vi "DP-Coerce Frequency.vi"(9 "Npts":i32, 10 "Sampling rate (Hz)":dbl, 11 "Frequency (kHz)":dbl[](array[numeric])) -> (1 "Npts":i32, 2 "Sampling rate (Hz)":dbl, 3 "Coerced Frequency (kHz)":dbl[](array[numeric]))   [LabVIEW 2020]
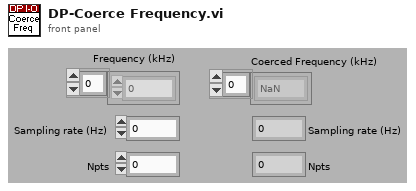
[diagram p1: front panel]
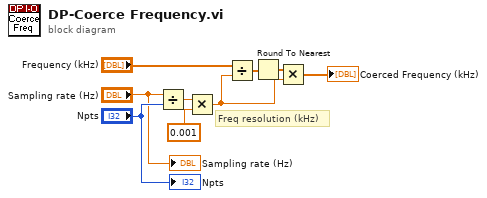
[diagram p0: block diagram]
diagram:
  # "Freq resolution (kHz)"
  n1 = Divide(x="Sampling rate (Hz)", y="Npts") -> (x/y=w9:dbl)
  n2 = Multiply(x=w9, y=0.001) -> (x*y=w6:dbl)
  n3 = Divide(x="Frequency (kHz)", y=w6) -> (x/y=w8:dbl[])
  n4 = Round To Nearest(number=w8) -> (nearest integer value=w7:dbl[])
  n5 = Multiply(x=w7, y=w6) -> (x*y=→"Coerced Frequency (kHz)":dbl[])
  "Sampling rate (Hz)" <- "Sampling rate (Hz)"
  "Npts" <- "Npts"
